vi "贪吃蛇.vi"() -> ()   [LabVIEW 2018]
panel:
  out "SR_REC":string
  out "GAME OVER":bool
  in  "速度":dbl(slide)=19.41747572815534 min=10.0 max=100.0 scale=0.0..100.0
  out "得分":i32
  in  "蛇":cluster{"X":i32, "Y":i32}[](array[cluster])
  in  "点":cluster{"X":i32, "Y":i32}={"X"=-1, "Y"=-1}
  in  "方向":enum16{"上", "下", "左", "右"}(ring)
  in  "运行":bool
  in  "退出":bool
  out "显示图":bool[][](array[boolean])
  # "声控贪吃蛇"
  # "语音控制 上下左右控制方向\n         单击开始游戏"
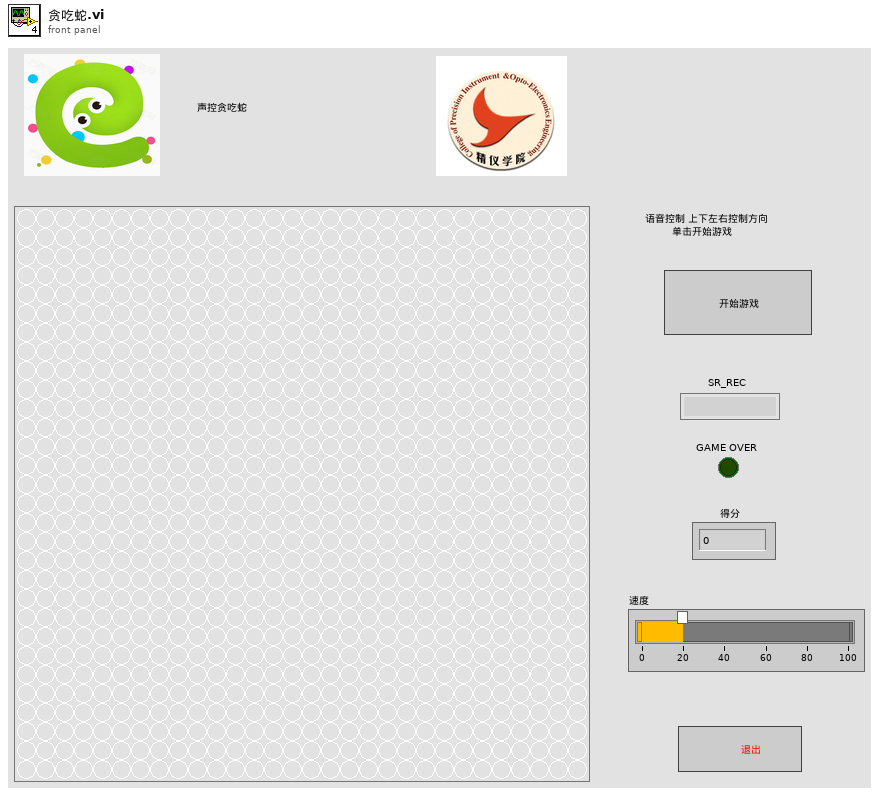
[diagram p1: front panel]
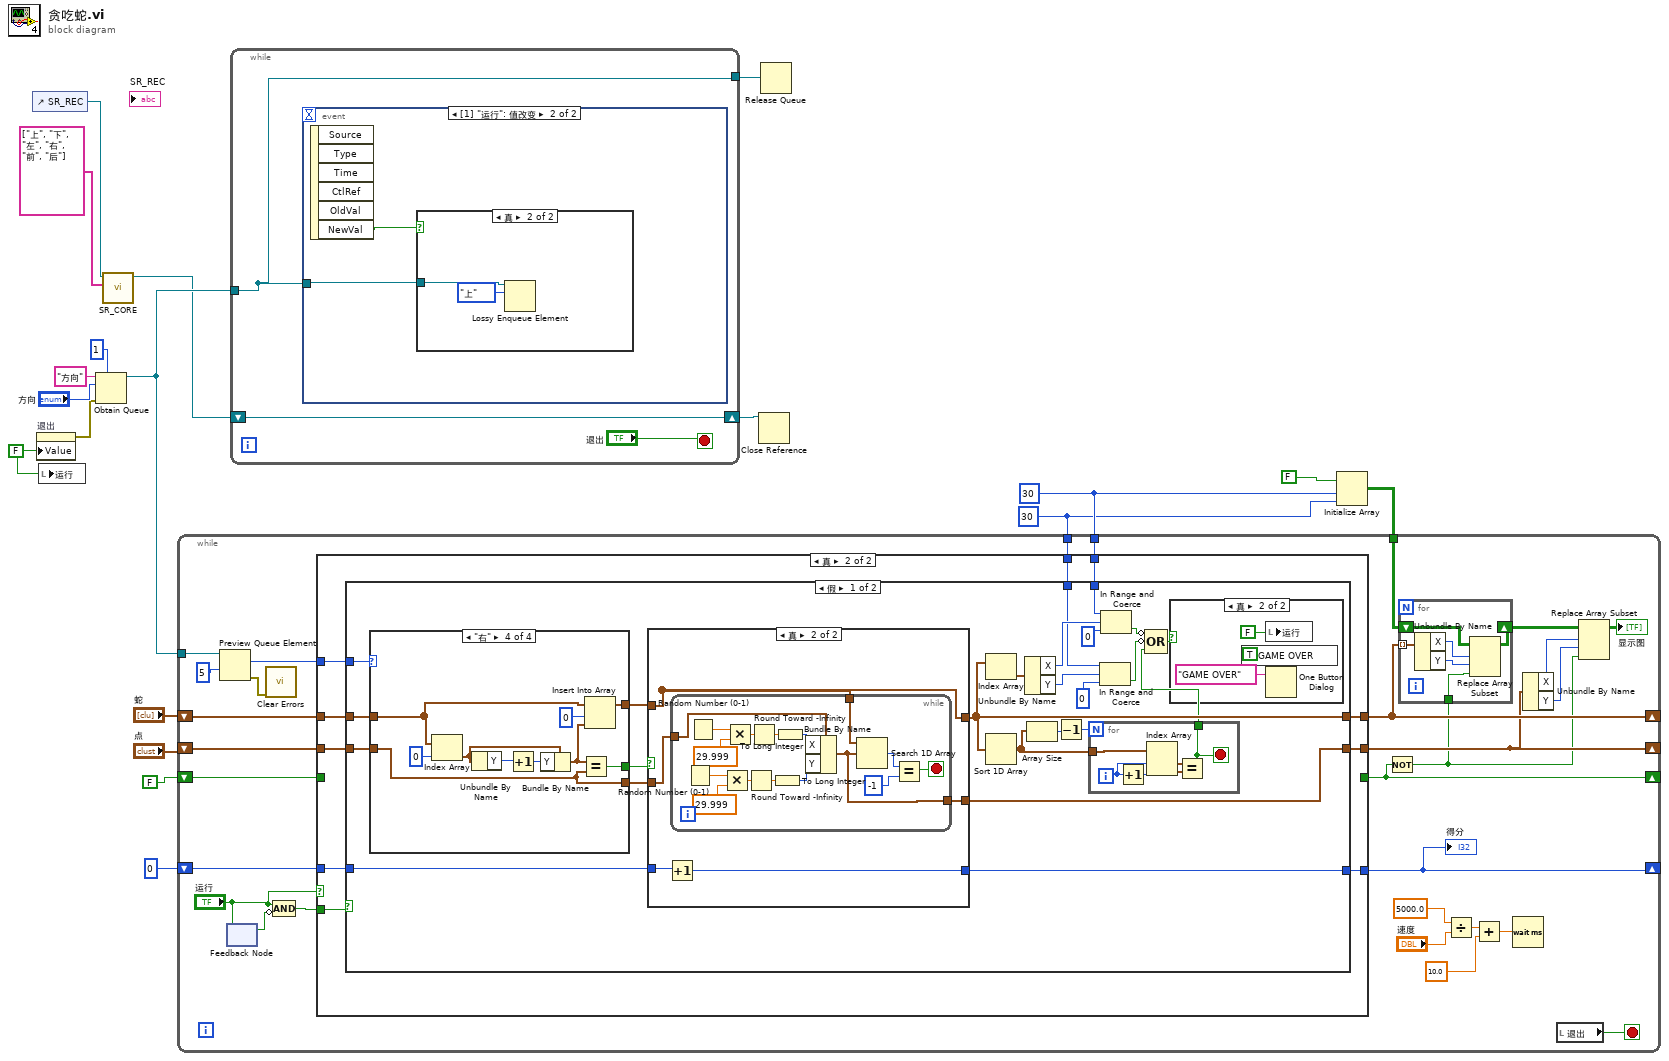
[diagram p0: block diagram]
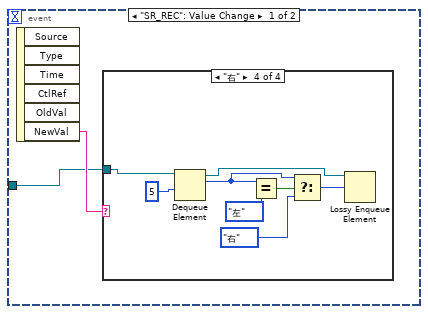
[diagram p2: hidden frame]
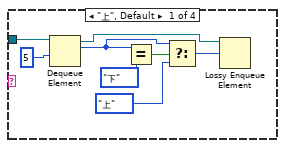
[diagram p3: hidden frame]
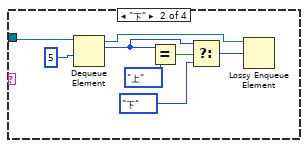
[diagram p4: hidden frame]
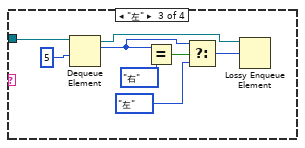
[diagram p5: hidden frame]
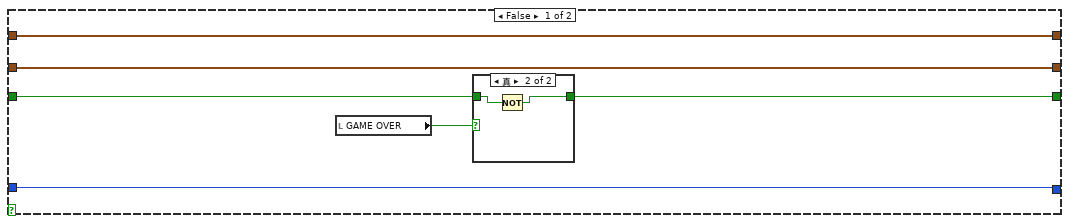
[diagram p7: hidden frame]
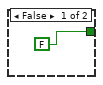
[diagram p8: hidden frame]
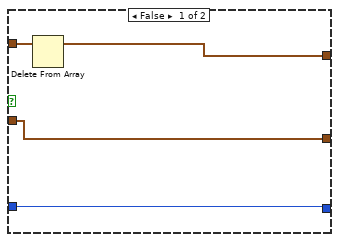
[diagram p10: hidden frame]
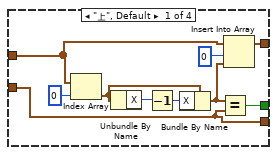
[diagram p11: hidden frame]
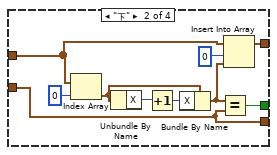
[diagram p12: hidden frame]
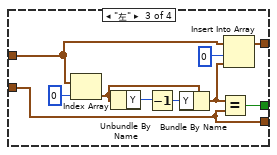
[diagram p13: hidden frame]
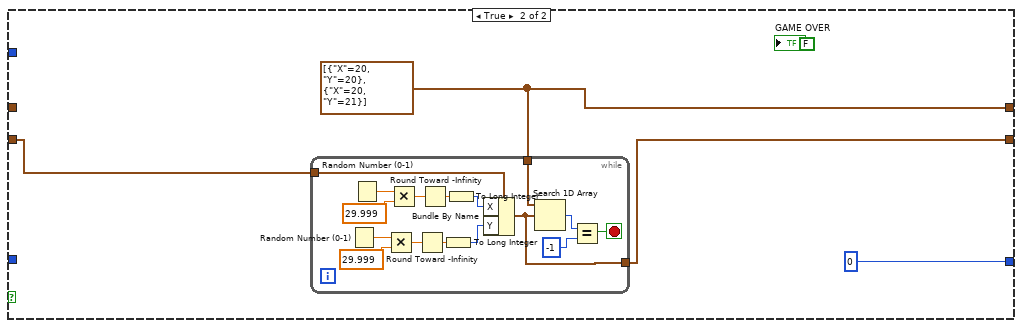
[diagram p14: hidden frame]
diagram:
  w6 = FALSE
  w9 = 30 ("维数大小")
  w10 = 30 ("维数大小")
  n1 = control-ref of="SR_REC"() -> (w3:refnum<vi>)
  n2 = property on="退出" class="Bool (严格)"("Value"=w6) -> (error out=w7:errorcluster)  [unwired: 2 in, 1 out]
  n3 = local write "运行"(w6) -> ()
  n4 = Obtain Queue(max queue size (-1, unlimited)=1, name (unnamed)="方向" ("名称（未命名）"), element data type="方向", error in (no error)=w7) -> (queue out=w13:refnum<queue>)  [unwired: 1 in, 2 out]
  n5 = call "SR_CORE.vi"("phrases"=string[] ["上", "下", "左", "右", "前", "后"], "SR_REC_TEXT"=w3) -> (".NET引用句柄输出"=w2:refnum<k24>)  [unwired: 8 in, 1 out]
  n6 = while {
    tunnel: w13 -> [w22]
    tunnel: [w22] -> w14
    shift-right: [w20] -> w1
    shift-left: w2 -> [w20]
    stop <- "退出" stop-if-true
    n7 = event shown="[1] \"运行\": 值改变" {
      selector: _ -> [_ _]
      dyn-events: _ -> [_ _]
      timeout: _ -> [_ _]
      tunnel: w22 -> [w23 w58]
      event "SR_REC": Value Change {
        n8 = event-data() -> ("NewVal"=w24:string)  [unwired: 1 in, 5 out]
        n9 = case shown="\"右\"" w24 {
          tunnel: w23 -> [w25 w33 w41 w49]
          frame "上", Default {
            n10 = Dequeue Element(queue=w25, timeout in ms (-1)=5) -> (queue out=w27:refnum<queue>, element=w28:enum16{"上", "下", "左", "右"})  [unwired: 1 in, 2 out]
            n11 = Equal?(x=w28, y=enum16{"上", "下", "左", "右"}."下") -> (x = y?=w30:bool)
            n12 = Select(t=w28, s=w30, f=enum16{"上", "下", "左", "右"}."上" ("y")) -> (s? t:f=w26:enum16{"上", "下", "左", "右"})
            n13 = Lossy Enqueue Element(queue=w27, element=w26) -> ()  [unwired: 1 in, 4 out]
          }
          frame "下" {
            n14 = Dequeue Element(queue=w33, timeout in ms (-1)=5) -> (queue out=w35:refnum<queue>, element=w36:enum16{"上", "下", "左", "右"})  [unwired: 1 in, 2 out]
            n15 = Equal?(x=w36, y=enum16{"上", "下", "左", "右"}."上") -> (x = y?=w38:bool)
            n16 = Select(t=w36, s=w38, f=enum16{"上", "下", "左", "右"}."下" ("y")) -> (s? t:f=w34:enum16{"上", "下", "左", "右"})
            n17 = Lossy Enqueue Element(queue=w35, element=w34) -> ()  [unwired: 1 in, 4 out]
          }
          frame "左" {
            n18 = Dequeue Element(queue=w41, timeout in ms (-1)=5) -> (queue out=w43:refnum<queue>, element=w44:enum16{"上", "下", "左", "右"})  [unwired: 1 in, 2 out]
            n19 = Equal?(x=w44, y=enum16{"上", "下", "左", "右"}."右") -> (x = y?=w46:bool)
            n20 = Select(t=w44, s=w46, f=enum16{"上", "下", "左", "右"}."左" ("y")) -> (s? t:f=w42:enum16{"上", "下", "左", "右"})
            n21 = Lossy Enqueue Element(queue=w43, element=w42) -> ()  [unwired: 1 in, 4 out]
          }
          frame "右" {
            n22 = Dequeue Element(queue=w49, timeout in ms (-1)=5) -> (queue out=w51:refnum<queue>, element=w52:enum16{"上", "下", "左", "右"})  [unwired: 1 in, 2 out]
            n23 = Equal?(x=w52, y=enum16{"上", "下", "左", "右"}."左") -> (x = y?=w54:bool)
            n24 = Select(t=w52, s=w54, f=enum16{"上", "下", "左", "右"}."右" ("y")) -> (s? t:f=w50:enum16{"上", "下", "左", "右"})
            n25 = Lossy Enqueue Element(queue=w51, element=w50) -> ()  [unwired: 1 in, 4 out]
          }
        }
      }
      event "运行": Value Change {
        n26 = event-data() -> ("NewVal"=w57:bool)  [unwired: 1 in, 5 out]
        n27 = case shown="真" w57 {
          tunnel: w58 -> [_ w60]
          frame False {
          }
          frame True {
            n28 = Lossy Enqueue Element(queue=w60, element=enum16{"上", "下", "左", "右"}."上" ("元素")) -> ()  [unwired: 1 in, 4 out]
          }
        }
      }
    }
  }
  n29 = Close Reference(reference=w1) -> ()  [unwired: 1 in, 1 out]
  n30 = Release Queue(queue=w14) -> ()  [unwired: 2 in, 3 out]
  n31 = Initialize Array(FALSE, w10, w9) -> (w18:bool[][])
  n32 = while {
    shift-right: [w84] -> _
    shift-left: "蛇" -> [w85]
    shift-right: [w81] -> _
    shift-left: "点" -> [w86]
    tunnel: w18 -> [w83]
    tunnel: w13 -> [w77]
    shift-right: [w73] -> _
    shift-left: 0 -> [w74]
    tunnel: w10 -> [w66]
    tunnel: w9 -> [w65]
    shift-right: [w63] -> _
    shift-left: FALSE -> [w64]
    stop <- w61 stop-if-true
    n33 = Preview Queue Element(queue=w77, timeout in ms (-1)=5) -> (element=w75:enum16{"上", "下", "左", "右"}, error out=w67:errorcluster)  [unwired: 1 in, 2 out]
    n34 = feedback-in #1("运行") -> ()
    n35 = feedback #1() -> (w89:bool)  [unwired: 1 in]
    n36 = call <vilib>:"Clear Errors.vi"("error in (no error)"=w67) -> ()  [unwired: 5 in, 2 out]
    n37 = Compound Arithmetic op=AND("运行", invert w89) -> (w88:bool)
    n38 = case shown="真" "运行" {
      tunnel: w88 -> [_ w114]
      tunnel: [w101 w113] -> w84
      tunnel: w86 -> [w99 w112]
      tunnel: [w99 w111] -> w81
      tunnel: w85 -> [w101 w110]
      tunnel: w75 -> [_ w109]
      tunnel: w74 -> [w100 w108]
      tunnel: [w100 w107] -> w73
      tunnel: w66 -> [_ w106]
      tunnel: w65 -> [_ w105]
      tunnel: w64 -> [w97 _]
      tunnel: [w96 _] -> w63
      frame False {
        n39 = local read "GAME OVER"() -> (w98:bool)
        n40 = case shown="真" w98 {
          tunnel: w97 -> [_ w104]
          tunnel: [FALSE w103] -> w96
          frame False {
          }
          frame True {
            n41 = Not(x=w104) -> (.not. x?=w103:bool)
          }
        }
      }
      frame True {
        n42 = case shown="假" w114 {
          tunnel: [w121 w216] -> w113
          tunnel: w112 -> [w137 w217]
          tunnel: [w133 w215] -> w111
          tunnel: w110 -> [w138 _]
          tunnel: w109 -> [w132 _]
          tunnel: w108 -> [w131 _]
          tunnel: [w130 0] -> w107
          tunnel: w106 -> [w120 _]
          tunnel: w105 -> [w119 _]
          frame False {
            n43 = case shown="\"右\"" w132 {
              tunnel: w138 -> [w180 w190 w200 w210]
              tunnel: [w175 w185 w195 w205] -> w134
              tunnel: w137 -> [w173 w183 w193 w203]
              tunnel: [w174 w184 w194 w204] -> w136
              tunnel: [w173 w183 w193 w203] -> w135
              frame "上", Default {
                n44 = Index Array(array=w180, index=0 ("索引 (行)")) -> (element=w179:cluster{"X":i32, "Y":i32})
                n45 = Unbundle By Name(w179) -> ("X"=w178:i32)
                n46 = Decrement(x=w178) -> (x-1=w177:i32)
                n47 = Bundle By Name(cluster=w179, "X"=w177) -> (w176:cluster{"X":i32, "Y":i32})
                n48 = Equal?(x=w176, y=w173) -> (x = y?=w174:bool)
                n49 = Insert Into Array(array=w180, index=0, new element=w176) -> (w175:cluster{"X":i32, "Y":i32}[])
              }
              frame "下" {
                n50 = Index Array(array=w190, index=0 ("索引 (行)")) -> (element=w189:cluster{"X":i32, "Y":i32})
                n51 = Unbundle By Name(w189) -> ("X"=w188:i32)
                n52 = Increment(x=w188) -> (x+1=w187:i32)
                n53 = Bundle By Name(cluster=w189, "X"=w187) -> (w186:cluster{"X":i32, "Y":i32})
                n54 = Equal?(x=w186, y=w183) -> (x = y?=w184:bool)
                n55 = Insert Into Array(array=w190, index=0, new element=w186) -> (w185:cluster{"X":i32, "Y":i32}[])
              }
              frame "左" {
                n56 = Index Array(array=w200, index=0 ("索引 (行)")) -> (element=w199:cluster{"X":i32, "Y":i32})
                n57 = Unbundle By Name(w199) -> ("Y"=w198:i32)
                n58 = Decrement(x=w198) -> (x-1=w197:i32)
                n59 = Bundle By Name(cluster=w199, "Y"=w197) -> (w196:cluster{"X":i32, "Y":i32})
                n60 = Equal?(x=w196, y=w193) -> (x = y?=w194:bool)
                n61 = Insert Into Array(array=w200, index=0, new element=w196) -> (w195:cluster{"X":i32, "Y":i32}[])
              }
              frame "右" {
                n62 = Index Array(array=w210, index=0 ("索引 (行)")) -> (element=w209:cluster{"X":i32, "Y":i32})
                n63 = Unbundle By Name(w209) -> ("Y"=w208:i32)
                n64 = Increment(x=w208) -> (x+1=w207:i32)
                n65 = Bundle By Name(cluster=w209, "Y"=w207) -> (w206:cluster{"X":i32, "Y":i32})
                n66 = Equal?(x=w206, y=w203) -> (x = y?=w204:bool)
                n67 = Insert Into Array(array=w210, index=0, new element=w206) -> (w205:cluster{"X":i32, "Y":i32}[])
              }
            }
            n68 = case shown="真" w136 {
              tunnel: w134 -> [w151 w156]
              tunnel: [w150 w156] -> w121
              tunnel: w135 -> [w149 w155]
              tunnel: [w149 w154] -> w133
              tunnel: w131 -> [w148 w153]
              tunnel: [w148 w152] -> w130
              frame False {
                n69 = Delete From Array(array=w151) -> (array with subset deleted=w150:cluster{"X":i32, "Y":i32}[])  [unwired: 2 in, 1 out]
              }
              frame True {
                n70 = Increment(x=w153) -> (x+1=w152:i32)
                n71 = while {
                  tunnel: w155 -> [w164]
                  tunnel: w156 -> [w161]
                  tunnel: [w157] -> w154
                  stop <- w158 stop-if-true
                  n72 = Random Number (0-1)() -> (number: 0 to 1=w165:dbl)
                  n73 = Random Number (0-1)() -> (number: 0 to 1=w172:dbl)
                  n74 = Multiply(x=w165, y=29.999) -> (x*y=w167:dbl)
                  n75 = Multiply(x=w172, y=29.999) -> (x*y=w170:dbl)
                  n76 = Round Toward -Infinity(1:w167) -> (0:w168:dbl)
                  n77 = Round Toward -Infinity(1:w170) -> (0:w169:dbl)
                  n78 = To Long Integer(number=w168) -> (32bit integer=w162:i32)
                  n79 = To Long Integer(number=w169) -> (32bit integer=w163:i32)
                  n80 = Bundle By Name(cluster=w164, "X"=w163, "Y"=w162) -> (w157:cluster{"X":i32, "Y":i32})
                  n81 = Search 1D Array(1D array=w161, element=w157) -> (index of element=w160:i32)  [unwired: 1 in]
                  n82 = Equal?(x=w160, y=-1) -> (x = y?=w158:bool)
                }
              }
            }
            n83 = Index Array(array=w121) -> (element=w129:cluster{"X":i32, "Y":i32})  [unwired: 1 in]
            n84 = Sort 1D Array(array=w121) -> (sorted array=w118:cluster{"X":i32, "Y":i32}[])
            n85 = Unbundle By Name(w129) -> ("X"=w128:i32, "Y"=w125:i32)
            n86 = Array Size(array=w118) -> (size(s)=w117:i32)
            n87 = Decrement(x=w117) -> (x-1=w116:i32)
            n88 = for {
              N: w116 -> [_]
              tunnel: w118 -> [w144]
              tunnel: [w139] -> w115
              i -> [w142]
              stop <- w139 stop-if-true
              n89 = Increment(x=w142) -> (x+1=w143:i32)
              n90 = Index Array(array=w144, index #1=w142, index #2=w143) -> (element #1=w141:cluster{"X":i32, "Y":i32}, element #2=w140:cluster{"X":i32, "Y":i32})
              n91 = Equal?(x=w141, y=w140) -> (x = y?=w139:bool)
            }
            n92 = In Range and Coerce(upper limit=w119, x=w125, lower limit=0 ("上限")) -> (In Range?=w123:bool)  [unwired: 1 out]
            n93 = In Range and Coerce(upper limit=w120, x=w128, lower limit=0 ("上限")) -> (In Range?=w124:bool)  [unwired: 1 out]
            n94 = Compound Arithmetic op=OR(invert w124, invert w123, w115) -> (w122:bool)
            n95 = case shown="真" w122 {
              frame False {
              }
              frame True {
                n96 = local write "GAME OVER"(TRUE) -> ()
                n97 = local write "运行"(FALSE) -> ()
                n98 = One Button Dialog(message="GAME OVER" ("消息")) -> ()  [unwired: 1 in, 1 out]
              }
            }
          }
          frame True {
            w216 = cluster{"X":i32, "Y":i32}[] [{"X"=20, "Y"=20}, {"X"=20, "Y"=21}] ("蛇")
            n99 = while {
              tunnel: w217 -> [w225]
              tunnel: w216 -> [w222]
              tunnel: [w218] -> w215
              stop <- w219 stop-if-true
              n100 = Random Number (0-1)() -> (number: 0 to 1=w226:dbl)
              n101 = Random Number (0-1)() -> (number: 0 to 1=w233:dbl)
              n102 = Multiply(x=w226, y=29.999) -> (x*y=w228:dbl)
              n103 = Multiply(x=w233, y=29.999) -> (x*y=w231:dbl)
              n104 = Round Toward -Infinity(1:w228) -> (0:w229:dbl)
              n105 = Round Toward -Infinity(1:w231) -> (0:w230:dbl)
              n106 = To Long Integer(number=w229) -> (32bit integer=w223:i32)
              n107 = To Long Integer(number=w230) -> (32bit integer=w224:i32)
              n108 = Bundle By Name(cluster=w225, "X"=w224, "Y"=w223) -> (w218:cluster{"X":i32, "Y":i32})
              n109 = Search 1D Array(1D array=w222, element=w218) -> (index of element=w221:i32)  [unwired: 1 in]
              n110 = Equal?(x=w221, y=-1) -> (x = y?=w219:bool)
            }
            "GAME OVER" <- FALSE
          }
        }
      }
    }
    "得分" <- w73
    n111 = Not(x=w63) -> (.not. x?=w62:bool)
    n112 = for {
      tunnel: w84 -> [w93] mode=indexing
      shift-right: [w94] -> w82
      shift-left: w83 -> [w95]
      tunnel: w62 -> [w90]
      n113 = Unbundle By Name(w93) -> ("X"=w92:i32, "Y"=w91:i32)
      n114 = Replace Array Subset(array=w95, new element=w90, index (row)=w92, index (col)=w91) -> (w94:bool[][])
    }
    n115 = Divide(x=5000.0, y="速度") -> (x/y=w70:dbl)
    n116 = Add(x=w70, y=10.0) -> (x+y=w69:dbl)
    n117 = Wait (ms)(milliseconds to wait=w69) -> ()  [unwired: 1 out]
    n118 = Unbundle By Name(w81) -> ("X"=w80:i32, "Y"=w79:i32)
    n119 = local read "退出"() -> (w61:bool)
    n120 = Replace Array Subset(array=w82, new element=w62, index (row)=w80, index (col)=w79) -> (→"显示图":bool[][])
  }
